vi "Add File.vi"(8 "error in (no error)":errorcluster, 9 "Insert in front":bool, 10 "File Path":path, 11 "Waveform Plot in":refnum<class "Waveform Plot.lvclass">) -> (0 "error out":errorcluster, 3 "Waveform Plot out":refnum<class "Waveform Plot.lvclass">)   [LabVIEW 2015, in "Waveform Plot.lvclass"]
uses:
  Waveform Plot.lvclass
  Plot/Plot.lvclass/Plot.ctl
  Plot/Write File-group-channel.vi
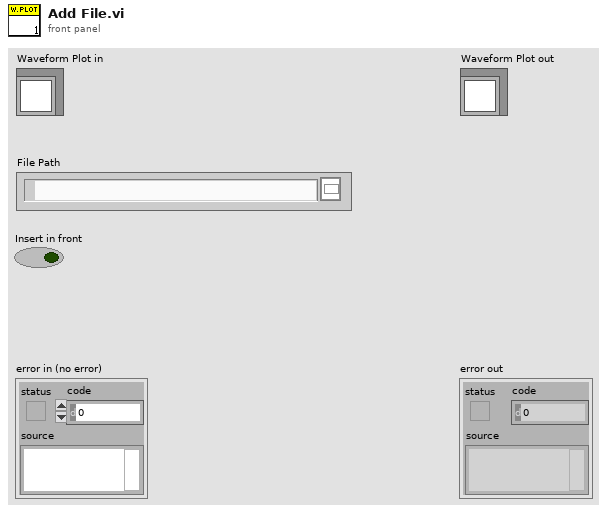
[diagram p1: front panel]
types:
  T1 = cluster{"File Path Control":path, "Group":string, "Channel":string, "Abbreviated":string}
  T2 = cluster{"File Path Control":path, "Group":string, "Channel":string, "Abbreviated":string}[]
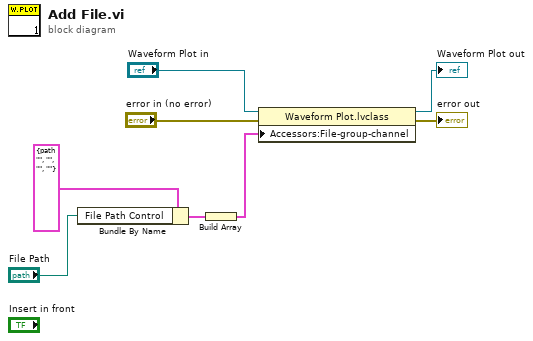
[diagram p0: block diagram]
diagram:
  n1 = Bundle By Name(cluster=T1 {"File Path Control"=path "", "Group"="", "Channel"="", "Abbreviated"=""} ("Cluster"), "File Path Control"="File Path") -> (w7:T1)
  n2 = Build Array(w7) -> (w8:T2)
  n3 = property class="Waveform Plot.lvclass"(reference="Waveform Plot in", error in="error in (no error)", "Accessors:File-group-channel"=w8) -> (reference out=→"Waveform Plot out":refnum<class "Waveform Plot.lvclass">, error out=→"error out":errorcluster)
